vi "generate_config_recorded_WFM.vi"(4 "Analog Out Channels":cluster{"0":bool, "1":bool}={"0"=TRUE, "1"=FALSE}, 5 "minimum value":dbl=-5.0, 6 "maximum value":dbl=5.0, 7 "path":path) -> (0 "error out":errorcluster, 1 "Sampling frequency(Hz)":dbl, 2 "signal Generated":waveform(dbl)(graph), 3 "task out":refnum<k21>)   [LabVIEW 2017]
uses:
  <vilib>/DAQmx/write.llb/DAQmx Write (Analog Wfm 1Chan NSamp).vi
  <vilib>/DAQmx/create/channels.llb/DAQmx Create Channel (AO-Voltage-Basic).vi
  <vilib>/Waveform/WDTOps.llb/WDT Append Waveforms DBL.vi
  <vilib>/DAQmx/configure/timing.llb/DAQmx Timing (Use Waveform).vi
  <vilib>/DAQmx/miscellaneous.llb/DAQmx Fill In Error Info.vi
  <instrlib>/NI USB-6356/NI USB-6356.lvlib
panel:
  out "size(s)":i32
  out "Number of channels":i32
  in  "error in":errorcluster
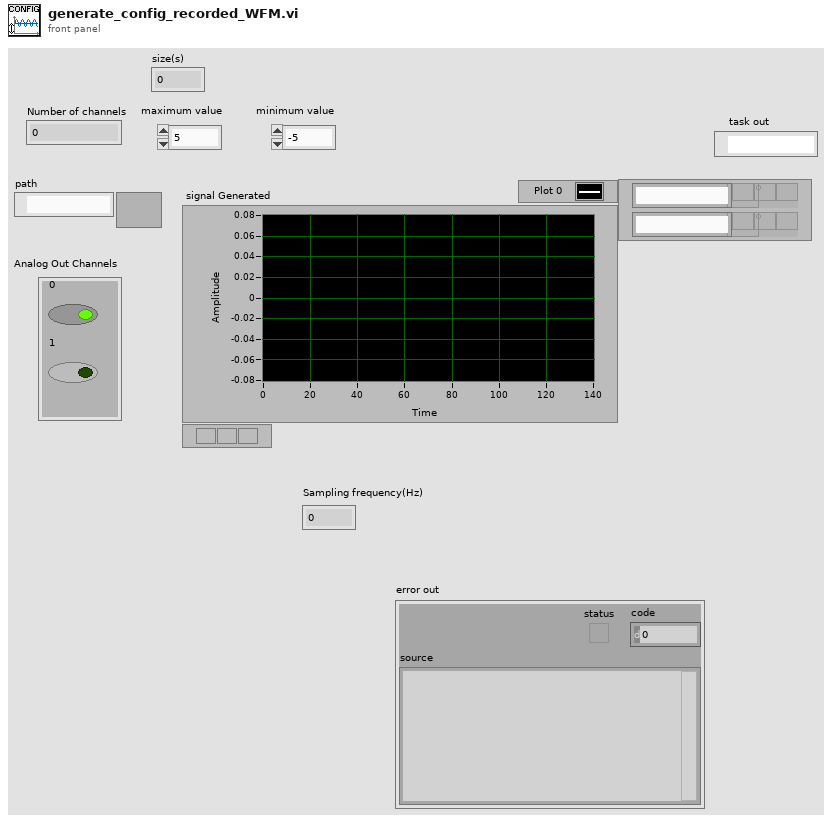
[diagram p1: front panel]
types:
  T1 = enum16{"open", "open or create", "create or replace", "create", "open (read-only)"}
  T2 = enum16{"Left Button", "Center Button", "Right Button", "Window Close"}
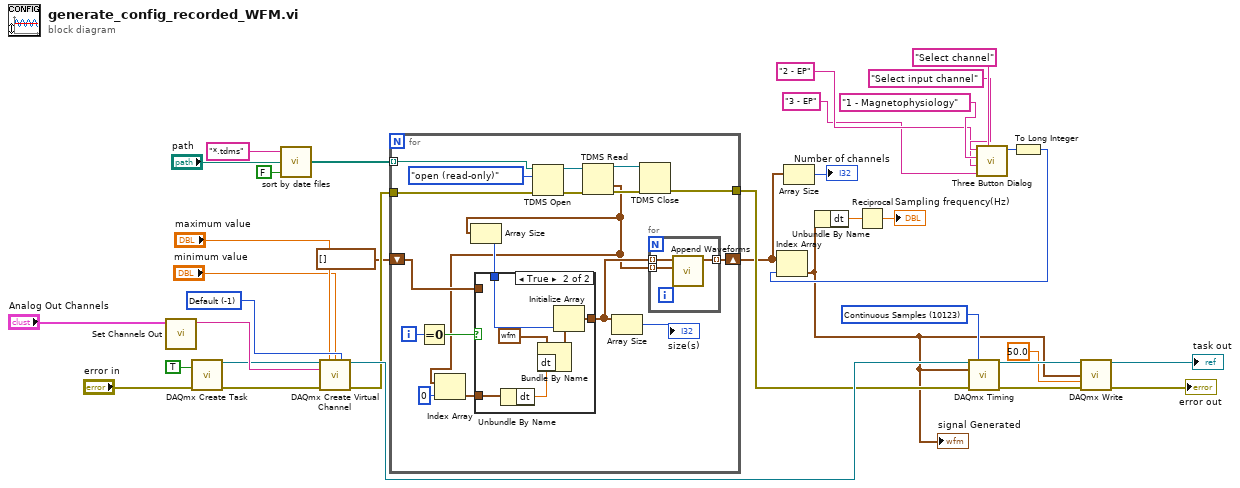
[diagram p0: block diagram]
diagram:
  w30 = 10123 items=["Finite Samples"=10178, "Continuous Samples"=10123, "Hardware Timed Single Point"=12522] ("sample mode")
  w35 = -1 items=["Default"=-1, "RSE"=10083, "Differential"=10106, "Pseudodifferential"=12529] ("output terminal configuration")
  n1 = call <instrlib>:"Set Channels Out.vi"("Analog Out Channels"="Analog Out Channels") -> ("String"=w34:string)  [unwired: 10 in]
  n2 = call <vilib>:"DAQmx Create Task.vi"("auto cleanup"=TRUE, "error in"="error in") -> ("task out"=w24:refnum<k21>, "error out"=w23:errorcluster)  [unwired: 12 in]
  n3 = call "sort by date files.vi"("Ascending (T) / Descending (F)"=FALSE, "path"="path", "pattern"="*.tdms") -> ("sorted list"=w16:path[])
  n4 = call-poly <vilib>:"DAQmx Create Virtual Channel.vi"("task in"=w24, "maximum value"="maximum value", "minimum value"="minimum value", "output terminal configuration"=w35, "physical channels"=w34, "error in"=w23) -> ("task out"=w33:refnum<k21>, "error out"=w15:errorcluster)  [unwired: 8 in]
  n5 = for {
    tunnel: w16 -> [w52] mode=indexing
    tunnel: w15 -> [w51]
    tunnel: [w48] -> w14
    shift-right: [w38] -> w1
    shift-left: waveform(dbl)[] [] -> [w42]
    i -> [w45]
    n6 = Equal To 0?(x=w45) -> (x = 0?=w44:bool)
    n7 = TDMS Open(8:w51, 10:T1."open (read-only)" ("operation (0:open)"), 11:w52) -> (0:w50:errorcluster, 3:w47:refnum<k34>)  [unwired: 4 in]
    n8 = TDMS Read(0:w47, 11:w50) -> (4:w46:refnum<k34>, 10:w37:waveform(dbl)[], 15:w49:errorcluster)  [unwired: 6 in, 3 out]
    n9 = Index Array(array=w37, index=0) -> (element=w36:waveform(dbl))
    n10 = Array Size(array=w37) -> (size(s)=w43:i32)
    n11 = case shown="True" w44 {
      tunnel: w43 -> [_ w60]
      tunnel: [w54 w59] -> w40
      tunnel: w42 -> [w54 _]
      tunnel: w36 -> [_ w57]
      frame False {
      }
      frame True {
        n12 = Unbundle By Name(w57) -> ("dt"=w55:dbl)
        n13 = Bundle By Name(cluster=waveform(dbl) {"t0"=timestamp(0 s since 1904-01-01), "dt"=1.0, "Y"=[]} ("Waveform"), "dt"=w55) -> (w56:waveform(dbl))
        n14 = Initialize Array(w56, w60) -> (w59:waveform(dbl)[])
      }
    }
    n15 = Array Size(array=w40) -> (size(s)=→"size(s)":i32)
    n16 = TDMS Close(8:w49, 11:w46) -> (0:w48:errorcluster)  [unwired: 1 out]
    n17 = for {
      tunnel: w37 -> [w63] mode=indexing
      tunnel: w40 -> [w62] mode=indexing
      tunnel: [w61] -> w38 mode=indexing
      n18 = call-poly <vilib>:"Append Waveforms.vi"("waveform B"=w63, "waveform A"=w62) -> ("waveform out"=w61:waveform(dbl))  [unwired: 8 in, 1 out]
    }
  }
  n19 = Array Size(array=w1) -> (size(s)=→"Number of channels":i32)
  n20 = call <vilib>:"Three Button Dialog.vi"("Window Title (\"\")"="Select channel" ("Window Title (\"\")"), "Right Button Text (\"Cancel\")"="3 - EP" ("message"), "Center Button Text (\"No\")"="2 - EP" ("message"), "Left Button Text (\"Yes\")"="1 - Magnetophysiology" ("message"), "message"="Select input channel") -> ("Which Button?"=w7:T2)  [unwired: 6 in]
  n21 = To Long Integer(number=w7) -> (32bit integer=w6:i32)
  n22 = Index Array(array=w1, index=w6) -> (element=w3:waveform(dbl))
  "signal Generated" <- w3
  n23 = Unbundle By Name(w3) -> ("dt"=w2:dbl)
  n24 = Reciprocal(x=w2) -> (1/x=→"Sampling frequency(Hz)":dbl)
  n25 = call-poly <vilib>:"DAQmx Timing.vi"("task/channels in"=w33, "sample mode"=w30, "waveform"=w3, "error in"=w14) -> ("task out"=w31:refnum<k21>, "error out"=w32:errorcluster)  [unwired: 10 in]
  n26 = call-poly <vilib>:"DAQmx Write.vi"("task/channels in"=w31, "data"=w3, "timeout"=50.0, "error in"=w32) -> ("task out"=→"task out":refnum<k21>, "error out"=→"error out":errorcluster)  [unwired: 9 in, 1 out]
